vi "parseDataI8Array.vi"(0 "U8ArrayParserAutoIndexing in":refnum<class "U8ArrayParserAutoIndexing.lvclass">, 1 "Length":i32, 3 "error in (no error)":errorcluster) -> (7 "U8ArrayParserAutoIndexing out":refnum<class "U8ArrayParserAutoIndexing.lvclass">, 8 "Data":i8[](array[numeric]), 10 "error out":errorcluster)   [LabVIEW 2016, in "RTUtilities.lvlib" / "U8ArrayParserAutoIndexing.lvclass"]
uses:
  U8ArrayParserAutoIndexing.lvclass
  U8ArrayParserAutoIndexing.lvclass/U8ArrayParserAutoIndexing.ctl
  U8ArrayParser/U8ArrayParserManualIndexing.lvclass
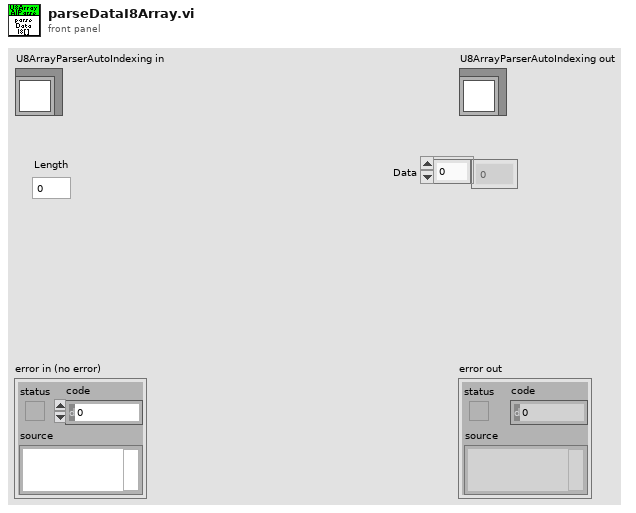
[diagram p1: front panel]
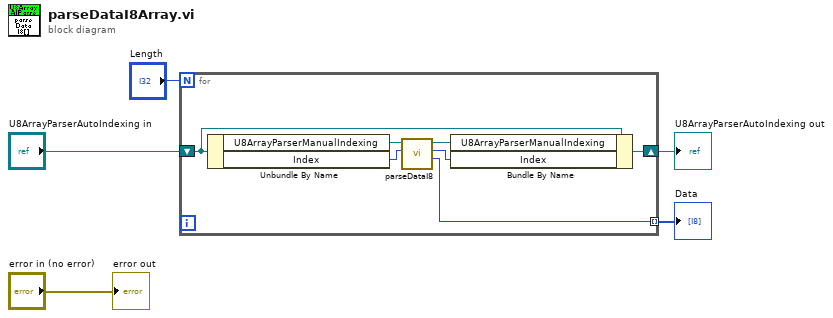
[diagram p0: block diagram]
diagram:
  n1 = for {
    N: "Length" -> [_]
    shift-right: [w7] -> w3
    shift-left: "U8ArrayParserAutoIndexing in" -> [w10]
    tunnel: [w6] -> w1 mode=indexing
    n2 = Unbundle By Name(w10) -> ("U8ArrayParserManualIndexing"=w12:refnum<class "U8ArrayParserManualIndexing.lvclass">, "Index"=w11:i32)
    n3 = call "parseDataI8.vi"("Index"=w11, "U8ArrayParserManualIndexing in"=w12) -> ("Data"=w6:i8, "Index out"=w8:i32, "U8ArrayParserManualIndexing out"=w9:refnum<class "U8ArrayParserManualIndexing.lvclass">)  [unwired: 6 in, 1 out]
    n4 = Bundle By Name(cluster=w10, "U8ArrayParserManualIndexing"=w9, "Index"=w8) -> (w7:refnum<class "U8ArrayParserAutoIndexing.lvclass">)
  }
  "U8ArrayParserAutoIndexing out" <- w3
  "Data" <- w1
  "error out" <- "error in (no error)"
